vi "Uint64Array Create (Dimensions).vi"(8 "error in (no error)":errorcluster, 10 "Array dimensions":i32[](array[numeric]), 11 "U64 array in":u64[](array[numeric])) -> (0 "error out":errorcluster, 3 "Uint64Array DVR out":refnum<data-value>)   [LabVIEW 2012, in "MDSplus.lvlib"]
uses:
  <vilib>/MDSplus/Library/MDSplus.lvlib
  <vilib>/MDSplus/Classes/Data_Class/Array_Class/Uint64Array_Class/Uint64Array.lvclass
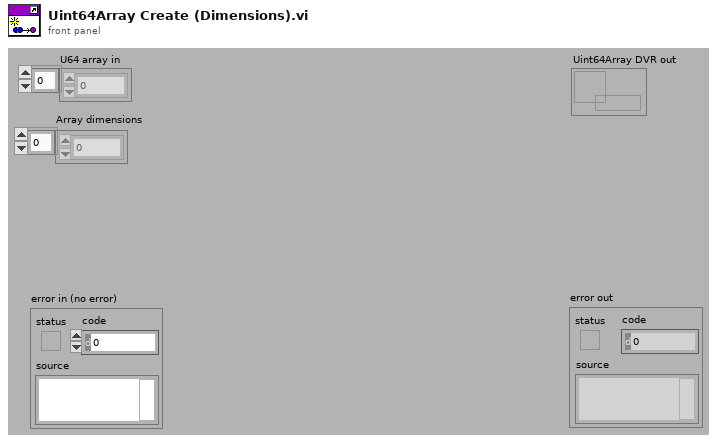
[diagram p1: front panel]
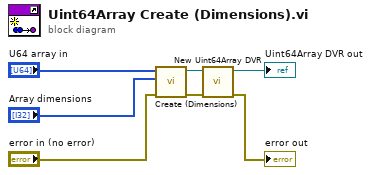
[diagram p0: block diagram]
diagram:
  n1 = call <vilib>:"Create (Dimensions).vi"("error in (no error)"="error in (no error)", "Dimensions"="Array dimensions", "U64 array in"="U64 array in") -> ("error out"=w4:errorcluster, "Uint64Array out"=w5:refnum<class "Uint64Array.lvclass">)  [unwired: 7 in]
  n2 = call <vilib>:"New Uint64Array DVR.vi"("error in (no error)"=w4, "Uint64Array in"=w5) -> ("error out"=→"error out":errorcluster, "Uint64Array DVR out"=→"Uint64Array DVR out":refnum<data-value>)  [unwired: 8 in]
